vi "Parse Smart Syntax Representation.vi"(0 "functionbase in":refnum<class "functionbase.lvclass">, 11 "error in (no error)":errorcluster) -> (4 "functionbase out":refnum<class "functionbase.lvclass">, 6 "Scan Syntax List":T1[](array[typedef]), 8 "Smart Syntax Representation List":string[](array[string]), 15 "error out":errorcluster)   [LabVIEW 2016, in "functionbase.lvclass"]
uses:
  functionbase.lvclass
  common/function utils/Scan Syntax Format.ctl
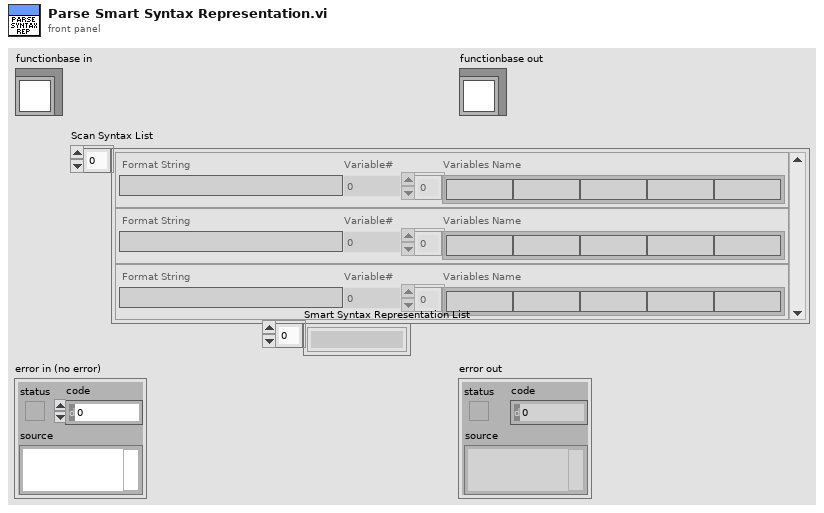
[diagram p1: front panel]
types:
  T1 = typedef "Scan Syntax Format.ctl" = cluster{"Format String":string, "Variable#":i32, "Variables Name":string[]}
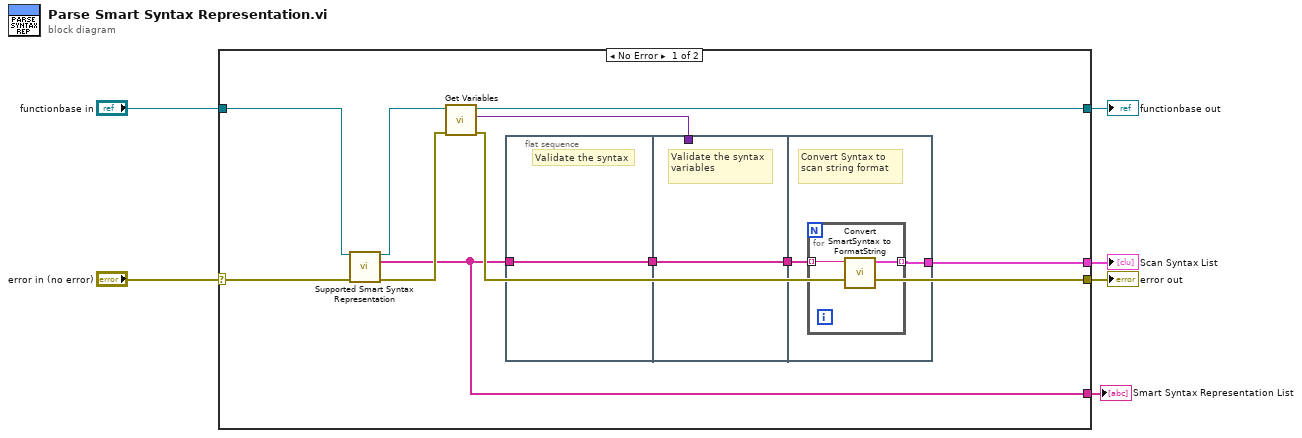
[diagram p0: block diagram]
diagram:
  n1 = case shown="No Error" "error in (no error)" {
    selector: "error in (no error)" -> [w16 w25]
    tunnel: [w14 w25] -> w5
    tunnel: [w12 w24] -> w3
    tunnel: "functionbase in" -> [w17 w24]
    tunnel: [w7 _] -> w2
    tunnel: [w8 _] -> w1
    frame No Error {
      n2 = call-dynamic "Supported Smart Syntax Representation.vi"("functionbase in"=w17, "error in (no error)"=w16) -> ("functionbase out"=w13:refnum<class "functionbase.lvclass">, "Smart Syntax Representation List"=w8:string[], "error out"=w15:errorcluster)  [unwired: 11 in]
      n3 = call-dynamic "Get Variables.vi"("error in (no error)"=w15, "functionbase in"=w13) -> ("error out"=w14:errorcluster, "Variables"=w10:variant, "functionbase out"=w12:refnum<class "functionbase.lvclass">)  [unwired: 7 in]
      n4 = flat-sequence {
        tunnel: w8 -> [w18]
        tunnel: [w18] -> w11
        tunnel: w11 -> [w19]
        tunnel: w10 -> [_]
        tunnel: [w19] -> w9
        tunnel: w9 -> [w21]
        tunnel: [w20] -> w7
        frame #0 {
          # "Validate the syntax"
        }
        frame #1 {
          # "Validate the syntax variables"
        }
        frame #2 {
          # "Convert Syntax to scan string format"
          n5 = for {
            tunnel: w21 -> [w23] mode=indexing
            tunnel: [w22] -> w20 mode=indexing
            n6 = call "Convert SmartSyntax to FormatString.vi"("Smart Syntax"=w23) -> ("Scan Syntax Format"=w22:T1)  [unwired: 9 in, 1 out]
          }
        }
      }
    }
    frame Error {
    }
  }
  "error out" <- w5
  "functionbase out" <- w3
  "Scan Syntax List" <- w2
  "Smart Syntax Representation List" <- w1
